vi "Get Parent Refnum if Invalid.vi"(8 "error in (no error)":errorcluster, 11 "VI Refnum In":refnum<vi>) -> (0 "error out":errorcluster, 2 "Invalid?":bool, 3 "VI Refnum Out":refnum<vi>)   [LabVIEW 2016, in "SLL Application.lvlib"]
uses:
  SLL Application.lvlib
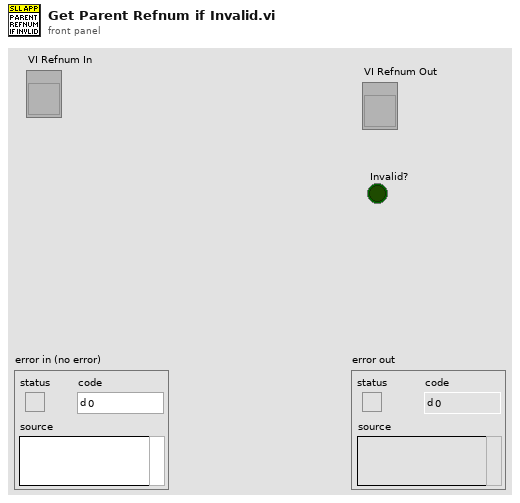
[diagram p1: front panel]
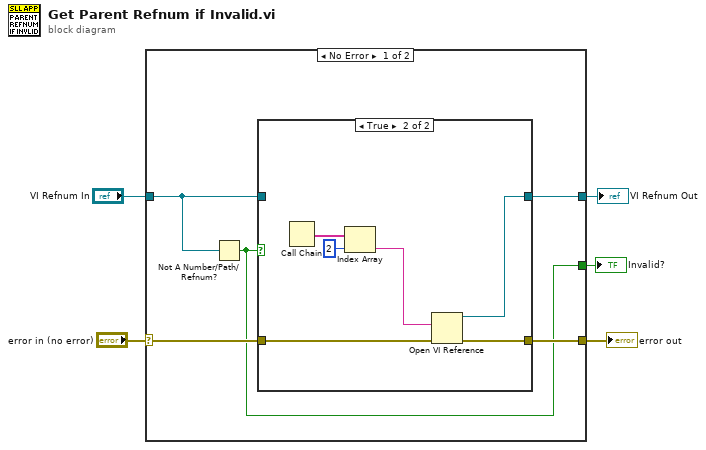
[diagram p0: block diagram]
diagram:
  n1 = case shown="No Error" "error in (no error)" {
    selector: "error in (no error)" -> [w10 w20]
    tunnel: [w9 w20] -> w4
    tunnel: "VI Refnum In" -> [w8 w19]
    tunnel: [w7 w19] -> w2
    tunnel: [w6 _] -> w1
    frame No Error {
      n2 = Not A Number/Path/Refnum?(number/path/refnum=w8) -> (NaN/Path/Refnum?=w6:bool)
      n3 = case shown="True" w6 {
        tunnel: w10 -> [w11 w16]
        tunnel: [w11 w15] -> w9
        tunnel: w8 -> [w12 _]
        tunnel: [w12 w13] -> w7
        frame False {
        }
        frame True {
          n4 = Call Chain() -> (call chain=w18:string[])
          n5 = Index Array(array=w18, index=2) -> (element=w14:string)
          n6 = Open VI Reference(vi path=w14, error in (no error)=w16) -> (vi reference=w13:refnum<vi>, error out=w15:errorcluster)  [unwired: 4 in]
        }
      }
    }
    frame Error {
    }
  }
  "error out" <- w4
  "VI Refnum Out" <- w2
  "Invalid?" <- w1
